vi "Pyramid_Path.vi"(4 "layers":dbl, 6 "height":dbl, 7 "vangle":dbl, 9 "width":dbl, 10 "increment":dbl, 11 "overlap":dbl) -> (3 "reference_corners":dbl[][](array[numeric]))   [LabVIEW 2015]
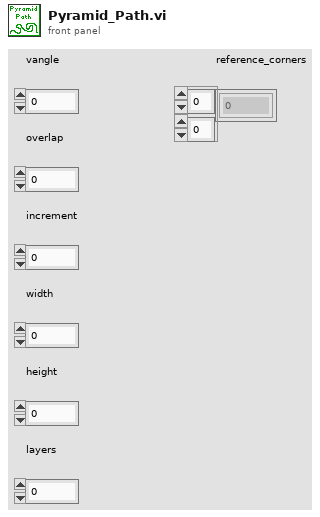
[diagram p1: front panel]
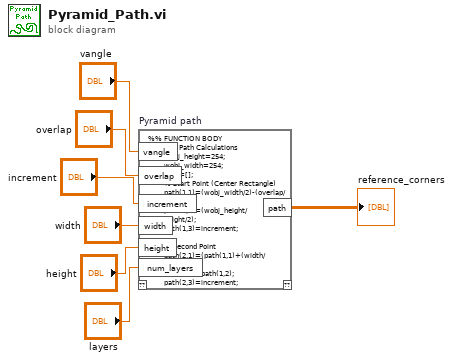
[diagram p0: block diagram]
diagram:
  n1 = script code="%% FUNCTION BODY    \n    %%% Path Calculations\n        wobj_height=254;\n        wobj_width=254;\n        path=[];\n        % Start Point (Center Rectangle)\n        path(1,1)=(wobj_width/2)-(overlap/2);\n        path(1,2)=(wobj_height/2)+(height/2);\n        path(1,3)=increment;\n        \n        % Second Point\n        path(2,1)=(path(1,1)+(width/2)+(overlap/2));\n        path(2,2)=path(1,2);\n        path(2,3)=increment;\n        \n        % Third Point\n        path(3,1)=path(2,1);\n        path(3,2)=(path(2,2)-height);\n        path(3,3)=increment;\n        \n        % Fourth Point\n        path(4,1)=(path(3,1)-width);\n        path(4,2)=path(3,2);\n        path(4,3)=increment;\n        \n        % Fifth Point\n        path(5,1)=path(4,1);\n        path(5,2)=(path(4,2)+height);\n        path(5,3)=increment;\n        \n        % Sixth Point\n        path(6,1)=(path(5,1)+(width/2)+(overlap/2));\n        path(6,2)=path(5,2);\n        path(6,3)=increment;\n        \n    % Path creation variables\n    layer_direction=-1;\n    current_point=7;\n    current_inc=2*increment;\n    length_offset=(increment*tan(vangle*(pi/180)));\n    current_length_offset=length_offset;\n    \n    % Layer incrementation\n    for i=2:num_layers\n        \n        %Point Calculations per each layer\n        for p=1:6\n            switch p\n                case 1\n                    % First Layer Point Calculations\n                    path(current_point,1)=(wobj_width/2)-(layer_direction*(overlap/2));\n                    path(current_point,2)=(wobj_height/2)+((height-(2*current_length_offset))/2);\n                case 2\n                    % Second Layer Point Calcuations\n                    path(current_point,1)=(path(current_point-1,1)+(layer_direction*(((width-(2*current_length_offset))/2)+(overlap/2))));\n                    path(current_point,2)=path(current_point-1,2);\n                case 3\n                    % Third Layer Point Calcuations\n                    path(current_point,1)=path(current_point-1,1);\n                    path(current_point,2)=(path(current_point-1,2)-(height-(2*current_length_offset)));\n                case 4\n                    % Fourth Layer Point Calcuations\n                    path(current_point,1)=(path(current_point-1,1)-(layer_direction*(width-(2*current_length_offset))));\n                    path(current_point,2)=path(current_point-1,2);\n                case 5\n                    % Fifth Layer Point Calcuations\n                    path(current_point,1)=path(current_point-1,1);\n                    path(current_point,2)=(path(current_point-1,2)+(height-(2*current_length_offset)));\n                case 6\n                    % Sixth Layer Point Calcuations\n                    path(current_point,1)=(path(current_point-1,1)+(layer_direction*(((width-(2*current_length_offset))/2)+(overlap/2))));\n                    path(current_point,2)=path(current_point-1,2);\n            end\n            % Data added to every point in a layer\n            path(current_point,3)=current_inc;\n            current_point=current_point+1;\n        end\n    %Index point offsets for next layer    \n    current_inc=current_inc+increment;\n    current_length_offset=current_length_offset+length_offset;\n    layer_direction=layer_direction*-1;\n    end\n    \n    %%% Approach/Retract Points\n        % Creates Approach Point\n        Approach_point=path(1,:);\n        Approach_point(3)=-50.8;\n    \n        % Creates Retract Point\n        Retract_point=path(end,:);\n        Retract_point(3)=-50.8;\n    \n        % Adds Approach/Retract Points to Path\n        path=[Approach_point',path',Retract_point',Approach_point'];\n        path=path';" "Pyramid path"("vangle"="vangle", "overlap"="overlap", "increment"="increment", "width"="width", "height"="height", "num_layers"="layers") -> ("path"=→"reference_corners":dbl[][])  [unwired: 1 in, 1 out]
